vi "Get Port CAN Cluster.vi"(8 "error in":errorcluster, 11 "Port Ref":T1 format="%.0x") -> (0 "error out":errorcluster, 2 "CAN Cluster":string, 3 "Port Ref out":T1 format="%.0x")   [LabVIEW 2020, in "Communication Bus Template Scripting.lvlib"]
uses:
  <vilib>/NI VeriStand/Custom Device API/Custom Device Item Ref.ctl
  Constants.vi
  Communication Bus Template Scripting.lvlib
  <vilib>/NI VeriStand/Custom Device API/Custom Device API.lvlib
  <vilib>/NI VeriStand/Custom Device API/Get Item Property (String).vi
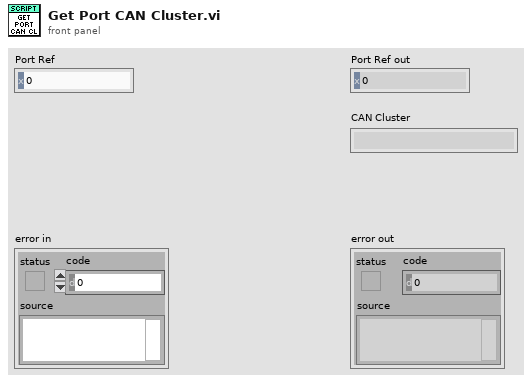
[diagram p1: front panel]
types:
  T1 = typedef "Custom Device API.lvlib/Custom Device Item Ref.ctl" = u64
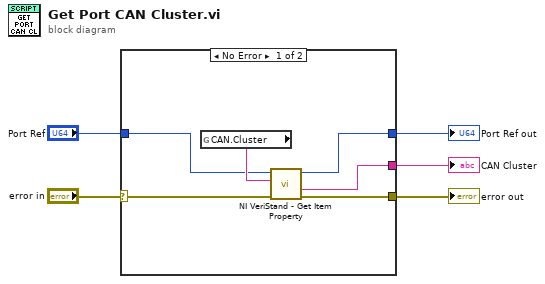
[diagram p0: block diagram]
diagram:
  n1 = case shown="No Error" "error in" {
    selector: "error in" -> [w7 w13]
    tunnel: "Port Ref" -> [w10 w12]
    tunnel: [w9 w13] -> w4
    tunnel: [w8 w12] -> w3
    tunnel: [w6 _] -> w1
    frame No Error {
      n2 = global read "Constants.vi" "CAN.Cluster"() -> (w11:string)
      n3 = call-poly <vilib>:"NI VeriStand - Get Item Property.vi"("error in (no error)"=w7, "Property Name"=w11, "Item Ref in"=w10) -> ("error out"=w9:errorcluster, "Value"=w6:string, "Item Ref out"=w8:T1)  [unwired: 5 in, 1 out]
    }
    frame Error {
    }
  }
  "error out" <- w4
  "CAN Cluster" <- w1
  "Port Ref out" <- w3
